vi "Sciospec_Control.vi"() -> ()   [LabVIEW 2012]
uses:
  <vilib>/Utility/file.llb/Write To Spreadsheet File (DBL).vi
  Sciospec ISX3 Impedance Analyzer.lvlib
panel:
  out "ACK for Start CMD 2":u8[](array[numeric])
  in  "MinutesToWait":dbl
  in  "Stop":bool
  out "Freq":dbl[](array[numeric])
  out "mag":dbl[](array[numeric])
  out "phase":dbl[](array[numeric])
  out "ACK for Start CMD":u8[](array[numeric])
  out "XY Graph 2":cluster{"Freq":dbl[], "phase":dbl[]}(graph)
  out "XY Graph":cluster{"Freq":dbl[], "mag":dbl[]}(graph)
  in  "Automatic Measurement":bool=TRUE
  out "Current Incoming row":u16
  out "SpecCount":u16
  in  "Number of Spectra":u16=1
  out "ACK for Set Channel":u8[](array[numeric])
  in  "Range Setting":u16(ring)=1 items=["100Ohm"=1, "10kOhm"=2, "1MOhm"=4]
  in  "Measurement Channel":u8(ring)=1 items=["BNC"=1, "ExtensionPort"=2, "ExtensionPort2"=3]
  in  "Save Slot":u8=1 min=1 step=1
  out "ACK for Save Setup":u8[](array[numeric])
  in  "Save Setup":bool
  out "ACK for Add Frequency":u8[](array[numeric])
  out "ACK for Init Setup":u8[](array[numeric])
  in  "Amplitude [V]":sgl=0.05 min=0.001 max=1
  in  "Precision":dbl=1.0 min=0.0
  in  "Frequency Count":sgl=101.0 min=1 max=2048 step=1
  in  "Stop Frequency [Hz]":sgl=1000000.0 min=0.1 max=1e+07
  in  "Start Frequency [Hz]":sgl=100.0 min=0.1 max=1e+07
  in  "Use LogScale":bool=TRUE
  # "Setup"
  # "Data Acquisition"
  # "Save the setup above"
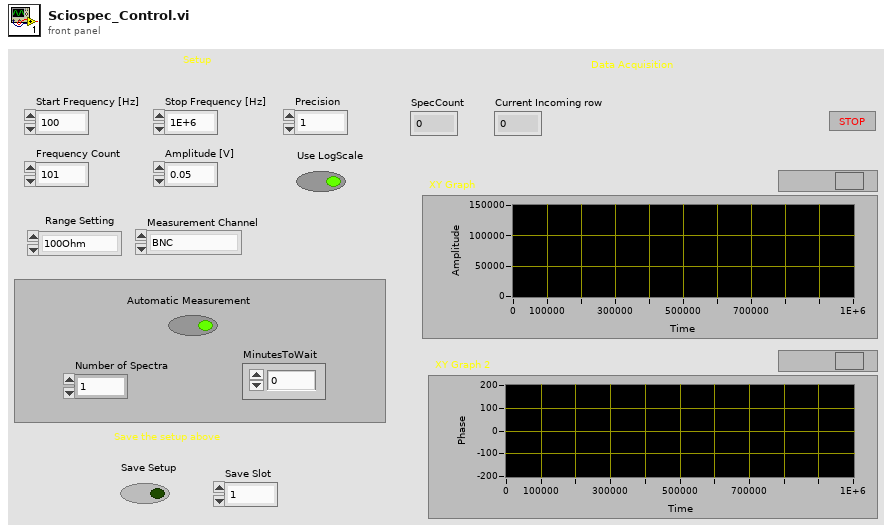
[diagram p1: front panel]
types:
  T1 = enum8{"Enabled", "Disabled", "Disabled and Grayed Out"}
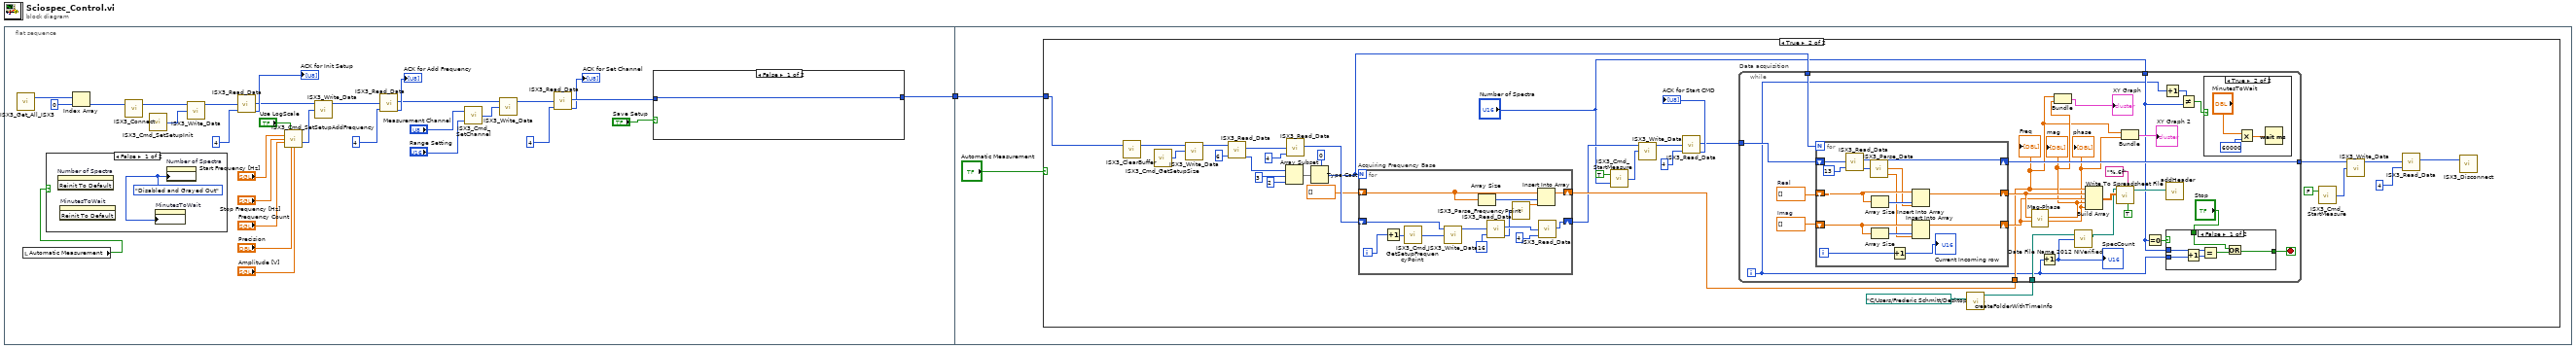
[diagram p0: block diagram]
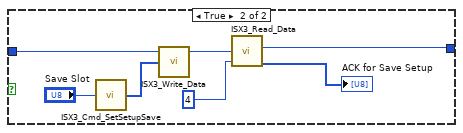
[diagram p3: hidden frame]
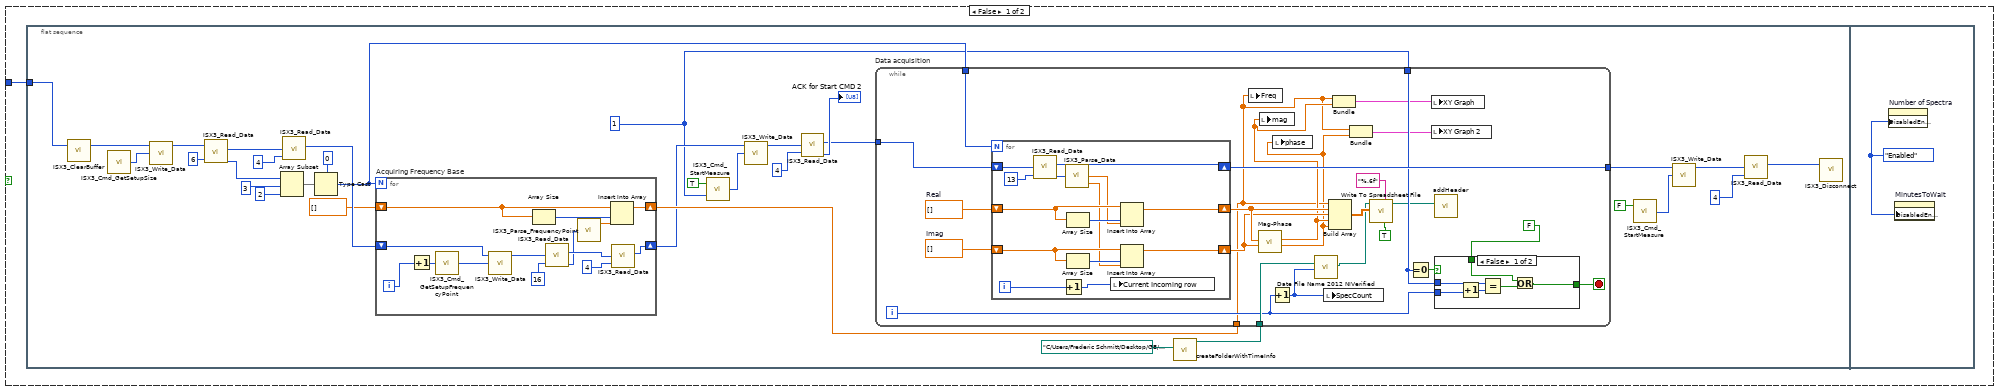
[diagram p4: hidden frame]
diagram:
  n1 = flat-sequence {
    tunnel: [w3] -> w1
    tunnel: w1 -> [w42]
    frame #0 {
      n2 = call "ISX3_Get_All_ISX3.vi"() -> ("A list of FT_Handel where an ISX-3 is connected to.\nThis handle must be used for further interaction \nwith the USB interface."=w16:u32[])  [unwired: 2 in]
      n3 = local read "Automatic Measurement"() -> (w2:bool)
      n4 = case shown="False" w2 {
        frame False {
          w32 = T1."Disabled and Grayed Out" ("Disabled")
          n5 = invoke on="Number of Spectra" class="DigNum (strict)" method="Reinit To Default"() -> ()  [unwired: 3 in, 3 out]
          n6 = invoke on="MinutesToWait" class="DigNum (strict)" method="Reinit To Default"() -> ()  [unwired: 3 in, 3 out]
          n7 = property on="MinutesToWait" class="DigNum (strict)"("DisabledEnum"=w32) -> ()  [unwired: 2 in, 2 out]
          n8 = property on="Number of Spectra" class="DigNum (strict)"("DisabledEnum"=w32) -> ()  [unwired: 2 in, 2 out]
        }
        frame True {
        }
      }
      n9 = Index Array(array=w16, index=u32 0) -> (element=w15:u32)
      n10 = call "ISX3_Connect.vi"("Connect to device with\nFT_Handle"=w15) -> ("Connected to device:"=w14:u32)  [unwired: 2 in]
      n11 = call "ISX3_Cmd_SetSetupInit.vi"() -> ("set Setup Init Cmd"=w12:u8[])  [unwired: 1 in]
      n12 = call "ISX3_Write_Data.vi"("Data to Write"=w12, "FT_Handle"=w14) -> ("FT_Handle"=w13:u32)  [unwired: 2 in, 1 out]
      n13 = call "ISX3_Read_Data.vi"("FT_Handle"=w13, "Bytes To Read"=4) -> ("Handle"=w10:u32, "Read Data"=→"ACK for Init Setup":u8[])  [unwired: 2 in, 1 out]
      n14 = call "ISX3_Cmd_SetSetupAddFrequency.vi"("Use LogScale"="Use LogScale", "Start Frequency [Hz]"="Start Frequency [Hz]", "Stop Frequency [Hz]"="Stop Frequency [Hz]", "Frequency Count"="Frequency Count", "Precision"="Precision", "Amplitude [V]"="Amplitude [V]") -> ("set Setup Init Cmd"=w11:u8[])  [unwired: 9 in]
      n15 = call "ISX3_Write_Data.vi"("Data to Write"=w11, "FT_Handle"=w10) -> ("FT_Handle"=w9:u32)  [unwired: 2 in, 1 out]
      n16 = call "ISX3_Read_Data.vi"("FT_Handle"=w9, "Bytes To Read"=4) -> ("Handle"=w6:u32, "Read Data"=→"ACK for Add Frequency":u8[])  [unwired: 2 in, 1 out]
      n17 = call "ISX3_Cmd_SetChannel.vi"("Range Setting"="Range Setting", "Measurement Channel"="Measurement Channel") -> ("set channel Cmd"=w5:u8[])
      n18 = call "ISX3_Write_Data.vi"("Data to Write"=w5, "FT_Handle"=w6) -> ("FT_Handle"=w4:u32)  [unwired: 2 in, 1 out]
      n19 = call "ISX3_Read_Data.vi"("FT_Handle"=w4, "Bytes To Read"=4) -> ("Handle"=w18:u32, "Read Data"=→"ACK for Set Channel":u8[])  [unwired: 2 in, 1 out]
      n20 = case shown="False" "Save Setup" {
        tunnel: w18 -> [w33 w36]
        tunnel: [w33 w39] -> w3
        frame False {
        }
        frame True {
          n21 = call "ISX3_Cmd_SetSetupSave.vi"("Setup Slot"="Save Slot") -> ("set Setup Save Cmd"=w35:u8[])
          n22 = call "ISX3_Write_Data.vi"("Data to Write"=w35, "FT_Handle"=w36) -> ("FT_Handle"=w34:u32)  [unwired: 2 in, 1 out]
          n23 = call "ISX3_Read_Data.vi"("FT_Handle"=w34, "Bytes To Read"=4) -> ("Handle"=w39:u32, "Read Data"=→"ACK for Save Setup":u8[])  [unwired: 2 in, 1 out]
        }
      }
    }
    frame #1 {
      n24 = case shown="True" "Automatic Measurement" {
        tunnel: w42 -> [w43 w136]
        frame False {
          n25 = flat-sequence {
            tunnel: w43 -> [w44]
            frame #0 {
              w54 = u16 1 ("Number of Spectra")
              n26 = call "ISX3_ClearBuffer.vi"("Handle"=w44) -> ("Handle"=w47:u32)  [unwired: 1 in, 1 out]
              n27 = call "ISX3_Cmd_GetSetupSize.vi"() -> ("get Setup Size Cmd"=w58:u8[])  [unwired: 1 in]
              n28 = call "ISX3_Write_Data.vi"("Data to Write"=w58, "FT_Handle"=w47) -> ("FT_Handle"=w59:u32)  [unwired: 2 in, 1 out]
              n29 = call "ISX3_Read_Data.vi"("FT_Handle"=w59, "Bytes To Read"=6) -> ("Handle"=w70:u32, "Read Data"=w68:u8[])  [unwired: 2 in, 1 out]
              n30 = Array Subset(array=w68, index=3, length=2) -> (w69:u8[])
              n31 = call "ISX3_Read_Data.vi"("FT_Handle"=w70, "Bytes To Read"=4) -> ("Handle"=w64:u32)  [unwired: 2 in, 2 out]
              n32 = Type Cast(type=u16 0, x=w69) -> (*(type *) &x=w61:u16)
              n33 = for "Acquiring Frequency Base" {
                N: w61 -> [_]
                shift-right: [w85] -> w63
                shift-left: dbl[] [] -> [w86]
                shift-right: [w82] -> w57
                shift-left: w64 -> [w80]
                i -> [w89]
                n34 = Increment(x=w89) -> (x+1=w81:i32)
                n35 = call "ISX3_Cmd_GetSetupFrequencyPoint.vi"("Row"=w81) -> ("get Setup Frequency Point Cmd"=w79:u8[])
                n36 = call "ISX3_Write_Data.vi"("Data to Write"=w79, "FT_Handle"=w80) -> ("FT_Handle"=w78:u32)  [unwired: 2 in, 1 out]
                n37 = Array Size(array=w86) -> (size(s)=w87:i32)
                n38 = call "ISX3_Read_Data.vi"("FT_Handle"=w78, "Bytes To Read"=16) -> ("Handle"=w84:u32, "Read Data"=w77:u8[])  [unwired: 2 in, 1 out]
                n39 = call "ISX3_Parse_FrequencyPoint.vi"("Array"=w77) -> ("Frequency [Hz]"=w76:sgl)  [unwired: 2 out]
                n40 = Insert Into Array(array=w86, index=w87, new element=w76) -> (w85:dbl[])
                n41 = call "ISX3_Read_Data.vi"("FT_Handle"=w84, "Bytes To Read"=4) -> ("Handle"=w82:u32)  [unwired: 2 in, 2 out]
              }
              n42 = call "ISX3_Cmd_StartMeasure.vi"("Number of Spectra"=w54, "Start/Stop"=TRUE) -> ("Start/Stop measurement cmd"=w53:u8[])
              n43 = call "ISX3_Write_Data.vi"("Data to Write"=w53, "FT_Handle"=w57) -> ("FT_Handle"=w56:u32)  [unwired: 2 in, 1 out]
              n44 = call "ISX3_Read_Data.vi"("FT_Handle"=w56, "Bytes To Read"=4) -> ("Handle"=w73:u32, "Read Data"=→"ACK for Start CMD 2":u8[])  [unwired: 2 in, 1 out]
              n45 = call "createFolderWithTimeInfo.vi"("Folder to save file to"=path "C:/Users/Frederic Schmitt/Desktop/GE/Sciospec Bioimpedance - Sinan/Sciospec ISX3v2/Data from LabVIEW") -> ("created path"=w46:path)  [unwired: 10 in]
              n46 = while "Data acquisition" {
                tunnel: w73 -> [w113]
                tunnel: [w110] -> w50
                tunnel: w63 -> [w93]
                tunnel: w54 -> [w108]
                tunnel: w61 -> [w106]
                tunnel: w46 -> [w102]
                i -> [w97]
                stop <- w107 stop-if-true
                w111 = dbl[] []  # Imag
                w112 = dbl[] []  # Real
                n47 = for {
                  N: w106 -> [_]
                  shift-right: [w133] -> w110
                  shift-left: w113 -> [w134]
                  shift-right: [w128] -> w100
                  shift-left: w112 -> [w126]
                  shift-right: [w130] -> w99
                  shift-left: w111 -> [w131]
                  i -> [w125]
                  n48 = call "ISX3_Read_Data.vi"("FT_Handle"=w134, "Bytes To Read"=13) -> ("Handle"=w133:u32, "Read Data"=w122:u8[])  [unwired: 2 in, 1 out]
                  n49 = Increment(x=w125) -> (x+1=w121:i32)
                  n50 = call "ISX3_Parse_Data.vi"("Array"=w122) -> ("Real"=w124:sgl, "Imag"=w123:sgl)  [unwired: 1 out]
                  n51 = Array Size(array=w126) -> (size(s)=w129:i32)
                  n52 = Array Size(array=w131) -> (size(s)=w132:i32)
                  n53 = local write "Current Incoming row"(w121) -> ()
                  n54 = Insert Into Array(array=w126, index=w129, new element=w124) -> (w128:dbl[])
                  n55 = Insert Into Array(array=w131, index=w132, new element=w123) -> (w130:dbl[])
                }
                n56 = local write "Freq"(w93) -> ()
                n57 = call "Mag-Phase.vi"("Imag"=w99, "Re"=w100) -> ("phase"=w92:dbl[], "mag"=w95:dbl[])  [unwired: 7 in]
                n58 = local write "mag"(w95) -> ()
                n59 = Increment(x=w97) -> (x+1=w96:i32)
                n60 = local write "phase"(w92) -> ()
                n61 = call "Date File Name 2012 NIVerified.vi"("Data Count"=w96, "Folder to save file to"=w102) -> ("New file path"=w103:path)  [unwired: 9 in]
                n62 = local write "SpecCount"(w96) -> ()
                n63 = Build Array(w93, w100, w99, w95, w92) -> (w105:dbl[][])
                n64 = Bundle(w93, "mag"=w95) -> (w94:cluster{dbl[], "mag":dbl[]})  [unwired: 1 in]
                n65 = Bundle(w93, "phase"=w92) -> (w91:cluster{dbl[], "phase":dbl[]})  [unwired: 1 in]
                n66 = call-poly <vilib>:"Write To Spreadsheet File.vi"("transpose? (no:F)"=TRUE, "format (%.3f)"="%.6f", "2D data"=w105, "file path (dialog if empty)"=w103) -> ("new file path (Not A Path if cancelled)"=w101:path)  [unwired: 4 in]
                n67 = Equal To 0?(x=w108) -> (x = 0?=w109:bool)
                n68 = local write "XY Graph"(w94) -> ()
                n69 = local write "XY Graph 2"(w91) -> ()
                n70 = call "addHeader.vi"("file path (dialog if empty)"=w101) -> ()  [unwired: 11 in]
                n71 = case shown="False" w109 {
                  tunnel: w108 -> [w119 _]
                  tunnel: w97 -> [w118 _]
                  tunnel: [w116 w120] -> w107
                  tunnel: FALSE -> [w115 w120]
                  frame False {
                    n72 = Increment(x=w118) -> (x+1=w117:i32)
                    n73 = Equal?(x=w119, y=w117) -> (x = y?=w114:bool)
                    n74 = Or(x=w115, y=w114) -> (x .or. y?=w116:bool)
                  }
                  frame True {
                  }
                }
              }
              n75 = call "ISX3_Cmd_StartMeasure.vi"("Start/Stop"=FALSE) -> ("Start/Stop measurement cmd"=w51:u8[])  [unwired: 1 in]
              n76 = call "ISX3_Write_Data.vi"("Data to Write"=w51, "FT_Handle"=w50) -> ("FT_Handle"=w49:u32)  [unwired: 2 in, 1 out]
              n77 = call "ISX3_Read_Data.vi"("FT_Handle"=w49, "Bytes To Read"=4) -> ("Handle"=w48:u32)  [unwired: 2 in, 2 out]
              n78 = call "ISX3_Disconnect.vi"("FT_Handle"=w48) -> ()  [unwired: 2 in]
            }
            frame #1 {
              w135 = T1."Enabled" ("Disabled")
              n79 = property on="Number of Spectra" class="DigNum (strict)"("DisabledEnum"=w135) -> ()  [unwired: 2 in, 2 out]
              n80 = property on="MinutesToWait" class="DigNum (strict)"("DisabledEnum"=w135) -> ()  [unwired: 2 in, 2 out]
            }
          }
        }
        frame True {
          n81 = call "ISX3_ClearBuffer.vi"("Handle"=w136) -> ("Handle"=w140:u32)  [unwired: 1 in, 1 out]
          n82 = call "ISX3_Cmd_GetSetupSize.vi"() -> ("get Setup Size Cmd"=w150:u8[])  [unwired: 1 in]
          n83 = call "ISX3_Write_Data.vi"("Data to Write"=w150, "FT_Handle"=w140) -> ("FT_Handle"=w151:u32)  [unwired: 2 in, 1 out]
          n84 = call "ISX3_Read_Data.vi"("FT_Handle"=w151, "Bytes To Read"=6) -> ("Handle"=w162:u32, "Read Data"=w160:u8[])  [unwired: 2 in, 1 out]
          n85 = Array Subset(array=w160, index=3, length=2) -> (w161:u8[])
          n86 = call "ISX3_Read_Data.vi"("FT_Handle"=w162, "Bytes To Read"=4) -> ("Handle"=w156:u32)  [unwired: 2 in, 2 out]
          n87 = Type Cast(type=u16 0, x=w161) -> (*(type *) &x=w153:u16)
          n88 = for "Acquiring Frequency Base" {
            N: w153 -> [_]
            shift-right: [w177] -> w155
            shift-left: dbl[] [] -> [w178]
            shift-right: [w174] -> w149
            shift-left: w156 -> [w172]
            i -> [w181]
            n89 = Increment(x=w181) -> (x+1=w173:i32)
            n90 = call "ISX3_Cmd_GetSetupFrequencyPoint.vi"("Row"=w173) -> ("get Setup Frequency Point Cmd"=w171:u8[])
            n91 = call "ISX3_Write_Data.vi"("Data to Write"=w171, "FT_Handle"=w172) -> ("FT_Handle"=w170:u32)  [unwired: 2 in, 1 out]
            n92 = Array Size(array=w178) -> (size(s)=w179:i32)
            n93 = call "ISX3_Read_Data.vi"("FT_Handle"=w170, "Bytes To Read"=16) -> ("Handle"=w176:u32, "Read Data"=w169:u8[])  [unwired: 2 in, 1 out]
            n94 = call "ISX3_Parse_FrequencyPoint.vi"("Array"=w169) -> ("Frequency [Hz]"=w168:sgl)  [unwired: 2 out]
            n95 = Insert Into Array(array=w178, index=w179, new element=w168) -> (w177:dbl[])
            n96 = call "ISX3_Read_Data.vi"("FT_Handle"=w176, "Bytes To Read"=4) -> ("Handle"=w174:u32)  [unwired: 2 in, 2 out]
          }
          n97 = call "ISX3_Cmd_StartMeasure.vi"("Number of Spectra"="Number of Spectra", "Start/Stop"=TRUE) -> ("Start/Stop measurement cmd"=w146:u8[])
          n98 = call "ISX3_Write_Data.vi"("Data to Write"=w146, "FT_Handle"=w149) -> ("FT_Handle"=w148:u32)  [unwired: 2 in, 1 out]
          n99 = call "ISX3_Read_Data.vi"("FT_Handle"=w148, "Bytes To Read"=4) -> ("Handle"=w165:u32, "Read Data"=→"ACK for Start CMD":u8[])  [unwired: 2 in, 1 out]
          n100 = call "createFolderWithTimeInfo.vi"("Folder to save file to"=path "C:/Users/Frederic Schmitt/Desktop/GE/Sciospec Bioimpedance - Sinan/Sciospec ISX3v2/Data from LabVIEW") -> ("created path"=w139:path)  [unwired: 10 in]
          n101 = while "Data acquisition" {
            tunnel: w165 -> [w207]
            tunnel: [w204] -> w143
            tunnel: w155 -> [w188]
            tunnel: "Number of Spectra" -> [w183]
            tunnel: w153 -> [w201]
            tunnel: w139 -> [w197]
            i -> [w182]
            stop <- w202 stop-if-true
            w205 = dbl[] []  # Imag
            w206 = dbl[] []  # Real
            n102 = for {
              N: w201 -> [_]
              shift-right: [w230] -> w204
              shift-left: w207 -> [w231]
              shift-right: [w225] -> w195
              shift-left: w206 -> [w223]
              shift-right: [w227] -> w194
              shift-left: w205 -> [w228]
              i -> [w222]
              n103 = call "ISX3_Read_Data.vi"("FT_Handle"=w231, "Bytes To Read"=13) -> ("Handle"=w230:u32, "Read Data"=w219:u8[])  [unwired: 2 in, 1 out]
              n104 = call "ISX3_Parse_Data.vi"("Array"=w219) -> ("Real"=w221:sgl, "Imag"=w220:sgl)  [unwired: 1 out]
              n105 = Array Size(array=w223) -> (size(s)=w226:i32)
              n106 = Array Size(array=w228) -> (size(s)=w229:i32)
              n107 = Increment(x=w222) -> (x+1=→"Current Incoming row":i32)
              n108 = Insert Into Array(array=w223, index=w226, new element=w221) -> (w225:dbl[])
              n109 = Insert Into Array(array=w228, index=w229, new element=w220) -> (w227:dbl[])
            }
            n110 = call "Mag-Phase.vi"("Imag"=w194, "Re"=w195) -> ("phase"=w187:dbl[], "mag"=w191:dbl[])  [unwired: 7 in]
            "mag" <- w191
            "phase" <- w187
            n111 = Increment(x=w182) -> (x+1=w186:i32)
            "SpecCount" <- w186
            n112 = Bundle(w188, "mag"=w191) -> (→"XY Graph":cluster{dbl[], "mag":dbl[]})  [unwired: 1 in]
            n113 = call "Date File Name 2012 NIVerified.vi"("Data Count"=w186, "Folder to save file to"=w197) -> ("New file path"=w198:path)  [unwired: 9 in]
            n114 = Build Array(w188, w195, w194, w191, w187) -> (w200:dbl[][])
            n115 = call-poly <vilib>:"Write To Spreadsheet File.vi"("transpose? (no:F)"=TRUE, "format (%.3f)"="%.6f", "2D data"=w200, "file path (dialog if empty)"=w198) -> ("new file path (Not A Path if cancelled)"=w196:path)  [unwired: 4 in]
            n116 = Bundle(w188, "phase"=w187) -> (→"XY Graph 2":cluster{dbl[], "phase":dbl[]})  [unwired: 1 in]
            n117 = Equal To 0?(x=w183) -> (x = 0?=w203:bool)
            n118 = Increment(x=w182) -> (x+1=w185:i32)
            n119 = call "addHeader.vi"("file path (dialog if empty)"=w196) -> ()  [unwired: 11 in]
            n120 = case shown="False" w203 {
              tunnel: w183 -> [w216 _]
              tunnel: w182 -> [w215 _]
              tunnel: [w213 w217] -> w202
              tunnel: "Stop" -> [w212 w217]
              frame False {
                n121 = Increment(x=w215) -> (x+1=w214:i32)
                n122 = Equal?(x=w216, y=w214) -> (x = y?=w211:bool)
                n123 = Or(x=w212, y=w211) -> (x .or. y?=w213:bool)
              }
              frame True {
              }
            }
            n124 = Not Equal?(x=w185, y=w183) -> (x != y?=w184:bool)
            n125 = case shown="True" w184 {
              frame False {
              }
              frame True {
                n126 = Multiply(x="MinutesToWait", y=u32 60000) -> (x*y=w210:dbl)
                n127 = Wait (ms)(milliseconds to wait=w210) -> ()  [unwired: 1 out]
              }
            }
            "Freq" <- w188
          }
          n128 = call "ISX3_Cmd_StartMeasure.vi"("Start/Stop"=FALSE) -> ("Start/Stop measurement cmd"=w144:u8[])  [unwired: 1 in]
          n129 = call "ISX3_Write_Data.vi"("Data to Write"=w144, "FT_Handle"=w143) -> ("FT_Handle"=w142:u32)  [unwired: 2 in, 1 out]
          n130 = call "ISX3_Read_Data.vi"("FT_Handle"=w142, "Bytes To Read"=4) -> ("Handle"=w141:u32)  [unwired: 2 in, 2 out]
          n131 = call "ISX3_Disconnect.vi"("FT_Handle"=w141) -> ()  [unwired: 2 in]
        }
      }
    }
  }
